vi "Parse String.vi"(8 "error in (no error)":errorcluster, 10 "Input String":string, 11 "ConfigManager.Text.INI in":refnum<class "ConfigManager.Text.INI.lvclass">) -> (0 "error out":errorcluster, 1 "Content":T1[](array[typedef]), 2 "Keys":string[](array[string]), 3 "ConfigManager.Text.INI out":refnum<class "ConfigManager.Text.INI.lvclass">, 5 "Section":string[](array[string]))   [LabVIEW 2013, in "CfgManager.Text.lvlib" / "ConfigManager.Text.INI.lvclass"]
uses:
  ConfigManager.Text.INI.lvclass
  Manager.Text/Dictionary Payload -- cluster.ctl
  Manager.Text/ConfigManager.Text.lvclass
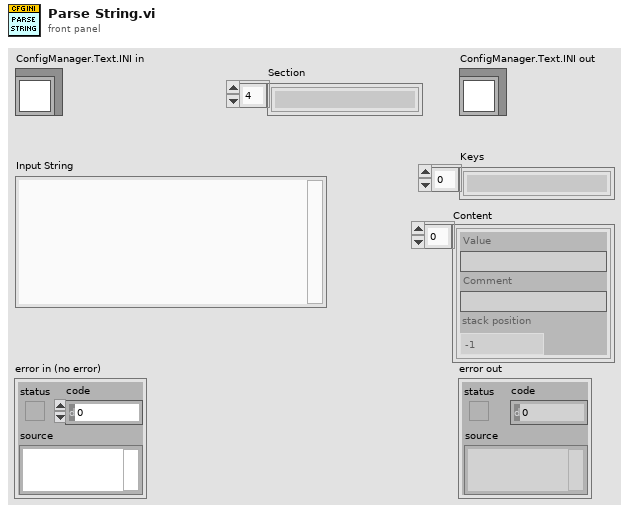
[diagram p1: front panel]
types:
  T1 = typedef "CfgManager.Text.lvlib/ConfigManager.Text.lvclass/Dictionary Payload -- cluster.ctl" = cluster{"Value":string, "Comment":string, "stack position":i32}
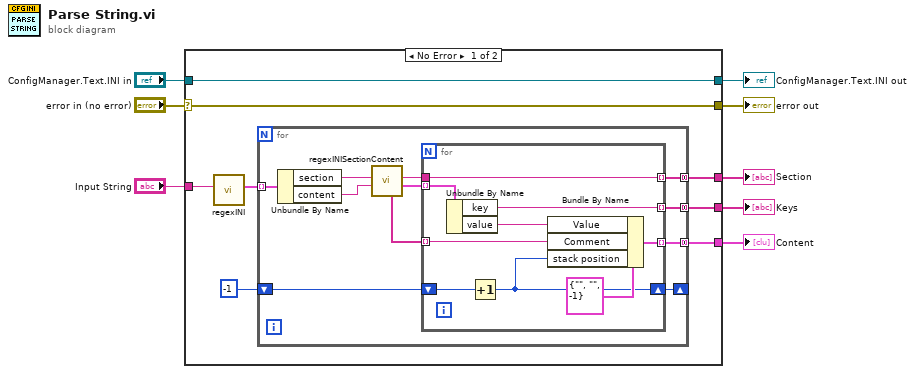
[diagram p0: block diagram]
diagram:
  n1 = case shown="No Error" "error in (no error)" {
    selector: "error in (no error)" -> [w16 w38]
    tunnel: [w16 w38] -> w7
    tunnel: [w15 w37] -> w5
    tunnel: "ConfigManager.Text.INI in" -> [w15 w37]
    tunnel: "Input String" -> [w14 _]
    tunnel: [w11 _] -> w3
    tunnel: [w10 _] -> w1
    tunnel: [w12 _] -> w2
    frame No Error {
      n2 = call "regexINI.vi"("INI String"=w14) -> ("Sections"=w13:cluster{"section":string, "content":string}[])  [unwired: 9 in, 1 out]
      n3 = for {
        tunnel: w13 -> [w27] mode=indexing
        tunnel: [w22] -> w12 mode=concatenating
        tunnel: [w21] -> w11 mode=concatenating
        tunnel: [w20] -> w10 mode=concatenating
        shift-right: [w17] -> _
        shift-left: -1 -> [w18]
        n4 = Unbundle By Name(w27) -> ("section"=w26:string, "content"=w25:string)
        n5 = call "regexINISectionContent.vi"("Section Content"=w25, "Section Name"=w26) -> ("KVPs"=w24:cluster{"key":string, "value":string}[], "Section Name dup"=w23:string, "Comments"=w19:string[])  [unwired: 6 in, 1 out]
        n6 = for {
          tunnel: w24 -> [w36] mode=indexing
          tunnel: w23 -> [w34]
          tunnel: [w35] -> w21 mode=indexing
          tunnel: [w30] -> w20 mode=indexing
          tunnel: [w34] -> w22 mode=indexing
          tunnel: w19 -> [w32] mode=indexing
          shift-right: [w28] -> w17
          shift-left: w18 -> [w29]
          n7 = Unbundle By Name(w36) -> ("key"=w35:string, "value"=w31:string)
          n8 = Increment(x=w29) -> (x+1=w28:i32)
          n9 = Bundle By Name(cluster=T1 {"Value"="", "Comment"="", "stack position"=-1} ("Dictionary Payload"), "Value"=w31, "Comment"=w32, "stack position"=w28) -> (w30:T1)
        }
      }
    }
    frame Error {
    }
  }
  "error out" <- w7
  "ConfigManager.Text.INI out" <- w5
  "Keys" <- w3
  "Content" <- w1
  "Section" <- w2
